vi "Benchmark - Transform And Project.vi"() -> ()   [LabVIEW 2020, in "Application.lvlib" / "Scene.lvclass"]
uses:
  Scene.lvclass
  ffc3b17b-87da-4396-a799-c2f73643b114.vi
  e688b912-8ed8-4bd5-a994-ea5027d429bc.vi
  Benchmark/Benchmark.lvlib
  <vilib>/Analysis/NI_AALBase.lvlib
panel:
  out "Std Dev":dbl format="%.1p"
  out "Mean":dbl format="%.1p"
  out "Histogram Graph":T1(graph)
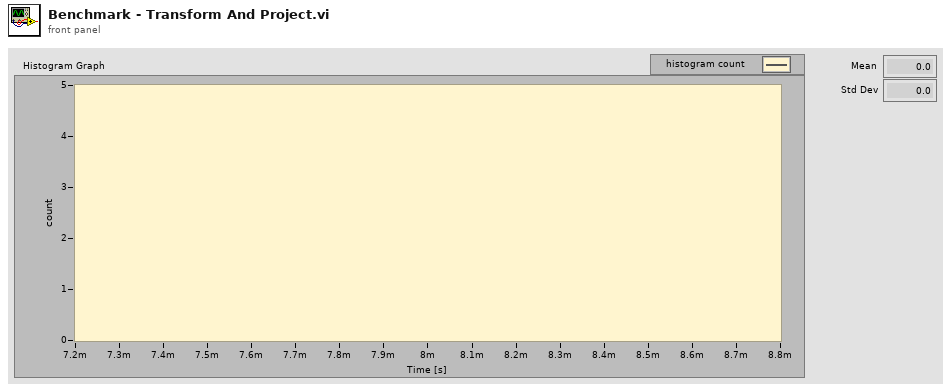
[diagram p1: front panel]
types:
  T1 = cluster{"X Values":dbl[], "Histogram: h(x)":i32[]}
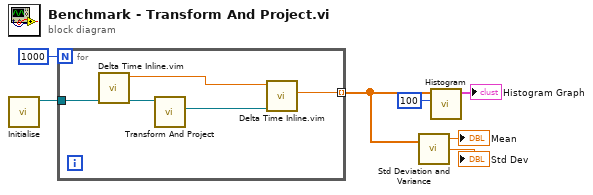
[diagram p0: block diagram]
diagram:
  n1 = call "Initialise.vi"() -> ("Scene out"=w1:refnum<class "Scene.lvclass">)  [unwired: 10 in, 1 out]
  n2 = for {
    N: 1000 -> [_]
    tunnel: [w12] -> w4 mode=indexing
    tunnel: w1 -> [w8]
    n3 = call "Delta Time Inline.vim"("value in"=w8) -> ("value out"=w9:refnum<class "Scene.lvclass">, "Relative Seconds out [s]"=w11:dbl)  [unwired: 8 in, 1 out]
    n4 = call "Transform And Project.vi"("Scene in"=w9) -> ("Scene out"=w10:refnum<class "Scene.lvclass">)  [unwired: 10 in]
    n5 = call "Delta Time Inline.vim"("value in"=w10, "Relative Seconds in [s]"=w11) -> ("Delta Time [s]"=w12:dbl)  [unwired: 7 in, 2 out]
  }
  n6 = call <vilib>:"Std Deviation and Variance.vi"("X"=w4) -> ("mean"=→"Mean":dbl, "standard deviation"=→"Std Dev":dbl)  [unwired: 1 in, 1 out]
  n7 = call <vilib>:"Histogram.vi"("intervals"=100, "X"=w4) -> ("Histogram Graph"=→"Histogram Graph":T1)  [unwired: 6 in, 3 out]
